vi "nominal run data source type at.vi"(8 "error in (no error)":errorcluster, 9 "out_type":i32, 10 "index":i32, 11 "run":i32) -> (0 "error out":errorcluster, 1 "out_type out":i32, 3 "function return":i32)   [LabVIEW 2020, in "client.lvlib"]
doc: "int32_t nominal_run_data_source_type_at(int32_t run, int32_t index, int32_t *out_type);"
uses:
  client.lvlib
  nominalClient_64.dll
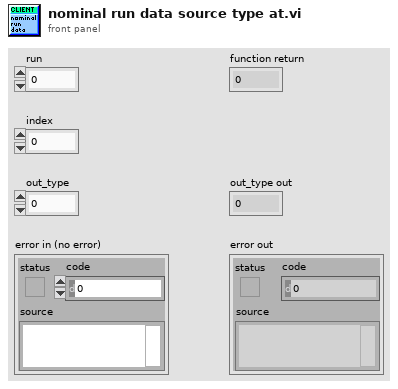
[diagram p1: front panel]
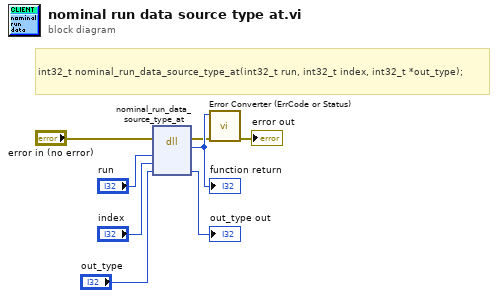
[diagram p0: block diagram]
diagram:
  # "int32_t nominal_run_data_source_type_at(int32_t run, int32_t index, int32_t *out_type);"
  n1 = dll-call lib="C:/code/labview-client-rs/lv_src/client/nominalClient_64.*" fn="nominal_run_data_source_type_at"(error in="error in (no error)", "run"="run", "index"="index", "out_type"="out_type") -> (error out=w2:errorcluster, w8:i32, "out_type"=→"out_type out":i32)  [unwired: 4 in, 1 out]
  "function return" <- w8
  n2 = call "Error Converter (ErrCode or Status).vi"("error in (no error)"=w2, "error code"=w8) -> ("error out"=→"error out":errorcluster)  [unwired: 9 in]
